vi "UpdateListBox.vi"(8 "error in (no error)":errorcluster, 10 "ListBox Refnum":refnum<vi>, 11 "9213 in":refnum<class "9213.lvclass">) -> (0 "error out":errorcluster, 3 "9213 out":refnum<class "9213.lvclass">)   [LabVIEW 2020, in "Modules.lvlib" / "9213.lvclass"]
uses:
  9213.lvclass
  <vilib>/Utility/miscctls.llb/LVRowAndColumnUnsignedTypeDef.ctl
  9213.lvclass/9213.ctl
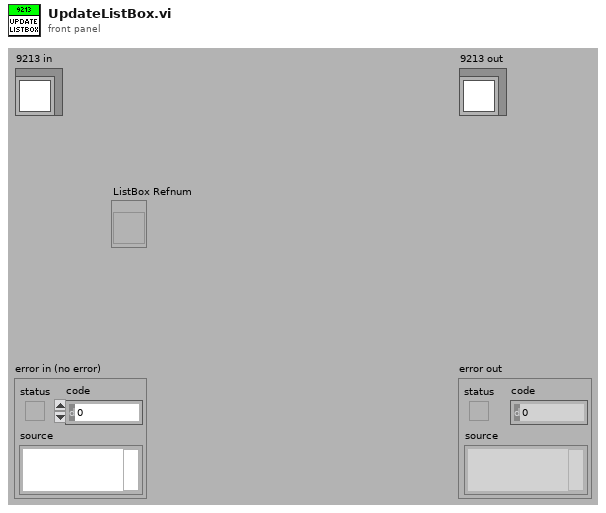
[diagram p1: front panel]
types:
  T1 = typedef "LVRowAndColumnUnsignedTypeDef.ctl" = cluster{"Row":u32, "Column":u32}
  T2 = typedef "Modules.lvlib/9213.lvclass/Thermocouple Type.ctl" = u8
  T3 = typedef "Modules.lvlib/9213.lvclass/Measurement Units.ctl" = u8
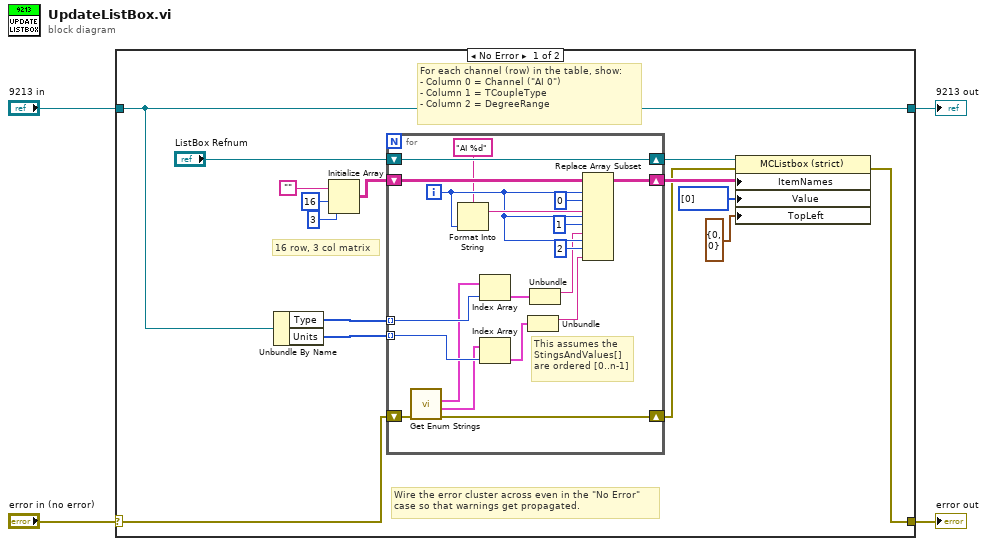
[diagram p0: block diagram]
diagram:
  n1 = case shown="No Error" "error in (no error)" {
    selector: "error in (no error)" -> [w9 w40]
    tunnel: [w7 w40] -> w3
    tunnel: [w10 w39] -> w1
    tunnel: "9213 in" -> [w10 w39]
    frame No Error {
      # "16 row, 3 col matrix"
      # "For each channel (row) in the table, show:\n- Column 0 = Channel (\"AI 0\")\n- Column 1 = TCoupleType\n- Column 2 = DegreeRange"
      # "Wire the error cluster across even in the \"No Error\"\ncase so that warnings get propagated."
      n2 = Unbundle By Name(w10) -> ("Type"=w17:T2[], "Units"=w16:T3[])
      n3 = Initialize Array("", 16 ("dimension size"), 3 ("dimension size")) -> (w14:string[][])
      n4 = for {
        shift-right: [w34] -> w19
        shift-left: w14 -> [w33]
        shift-right: [w38] -> w18
        shift-left: "ListBox Refnum" -> [w38]
        tunnel: w17 -> [w36] mode=indexing
        tunnel: w16 -> [w37] mode=indexing
        shift-right: [w20] -> w8
        shift-left: w9 -> [w21]
        i -> [w30]
        # "This assumes the StingsAndValues[] are ordered [0..n-1]"
        n5 = call "Get Enum Strings.vi"("error in (no error)"=w21) -> ("error out"=w20:errorcluster, "Units"=w22:cluster{"String":string, "Value":u16}[], "Type"=w23:cluster{"String":string, "Value":u16}[])  [unwired: 8 in]
        n6 = Format Into String(format string="AI %d", w30) -> (resulting string=w31:string)  [unwired: 2 in, 1 out]
        n7 = Index Array(array=w23, index=w36) -> (element=w28:cluster{"String":string, "Value":u16})
        n8 = Index Array(array=w22, index=w37) -> (element=w27:cluster{"String":string, "Value":u16})
        n9 = Unbundle(w27) -> ("String"=w24:string)  [unwired: 1 out]
        n10 = Unbundle(w28) -> ("String"=w25:string)  [unwired: 1 out]
        n11 = Replace Array Subset(array=w33, new element #1=w31, index (row) #1=w30, index (col) #1=0 ("Column 1"), new element #2=w25, index (row) #2=w30, index (col) #2=1 ("Column 1"), new element #3=w24, index (row) #3=w30, index (col) #3=2 ("disabled index (col)")) -> (w34:string[][])
      }
      n12 = property on="Property Node" class="MCListbox (strict)"(reference=w18, error in=w8, "ItemNames"=w19, "Value"=i32[] [0], "TopLeft"=T1 {"Row"=0, "Column"=0} ("Top Left Visible Cell")) -> (error out=w7:errorcluster)  [unwired: 1 out]
    }
    frame Error {
    }
  }
  "error out" <- w3
  "9213 out" <- w1
